vi "Add.vi"(6 "Options":T1={"DbType"=-1, "Direction"=-1, "Size"=-1, "Precision"=255, "Scale"=255} {"Direction" items=["Input"=1, "Output"=2, "InputOutput"=3, "ReturnValue"=6]; "DbType" items=["AnsiString"=0, "Binary"=1, "Byte"=2, "Boolean"=3, "Currency"=4, "Date"=5, "DateTime"=6, "Decimal"=7, "Double"=8, "Guid"=9, "Int16"=10, "Int32"=11, "Int64"=12, "Object"=13, "SByte"=14, "Single"=15, "String"=16, "Time"=17, "UInt16"=18, "UInt32"=19, "UInt64"=20, "VarNumeric"=21, "AnsiStringFixedLength"=22, "StringFixedLength"=23, "Xml"=25, "DateTime2"=26, "DateTimeOffset"=27]}, 8 "error in (no error)":errorcluster, 9 "value":variant, 10 "name":string, 11 "DynamicParameters in":refnum<class "DapperParameters.lvclass">) -> (0 "error out":errorcluster, 3 "DynamicParameters out":refnum<class "DapperParameters.lvclass">)   [LabVIEW 2020, in "ORM_Dapper.lvlib" / "DapperParameters.lvclass"]
uses:
  DapperParameters.lvclass
  System.Data
  DapperParameters.lvclass/DapperParameters.ctl
  C:/Viviota/Projects/R&D/__OpenSource/VIV_ORM/libraries/npgsql/System.Text.Json.dll
  libraries/npgsql/System.Text.Json.dll
  C:/Viviota/Projects/R&D/__OpenSource/VIV_ORM/libraries/dapper/Dapper.dll
  libraries/dapper/Dapper.dll
  Read ref.vi
  <vilib>/Viviota/shared/ORM.lvlibp/ORM/DynamicParameters/DynamicParameters.lvclass
  C:/Program Files/National Instruments/LabVIEW 2020/vi.lib/Viviota/shared/ORM.lvlibp/ORM/DynamicParameters/DynamicParameters.lvclass
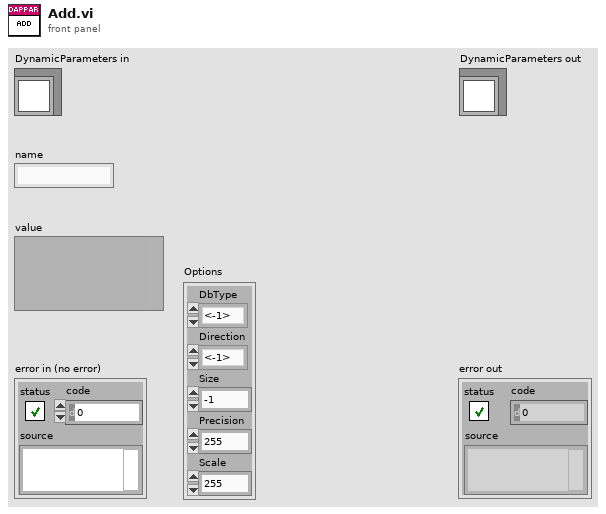
[diagram p1: front panel]
types:
  T1 = cluster{"DbType":i32, "Direction":i32, "Size":i32, "Precision":u8, "Scale":u8}
  T2 = typedef "ORM_Dapper.lvlib/dapper_dynamicparameters_ref.ctl" = refnum<k24>
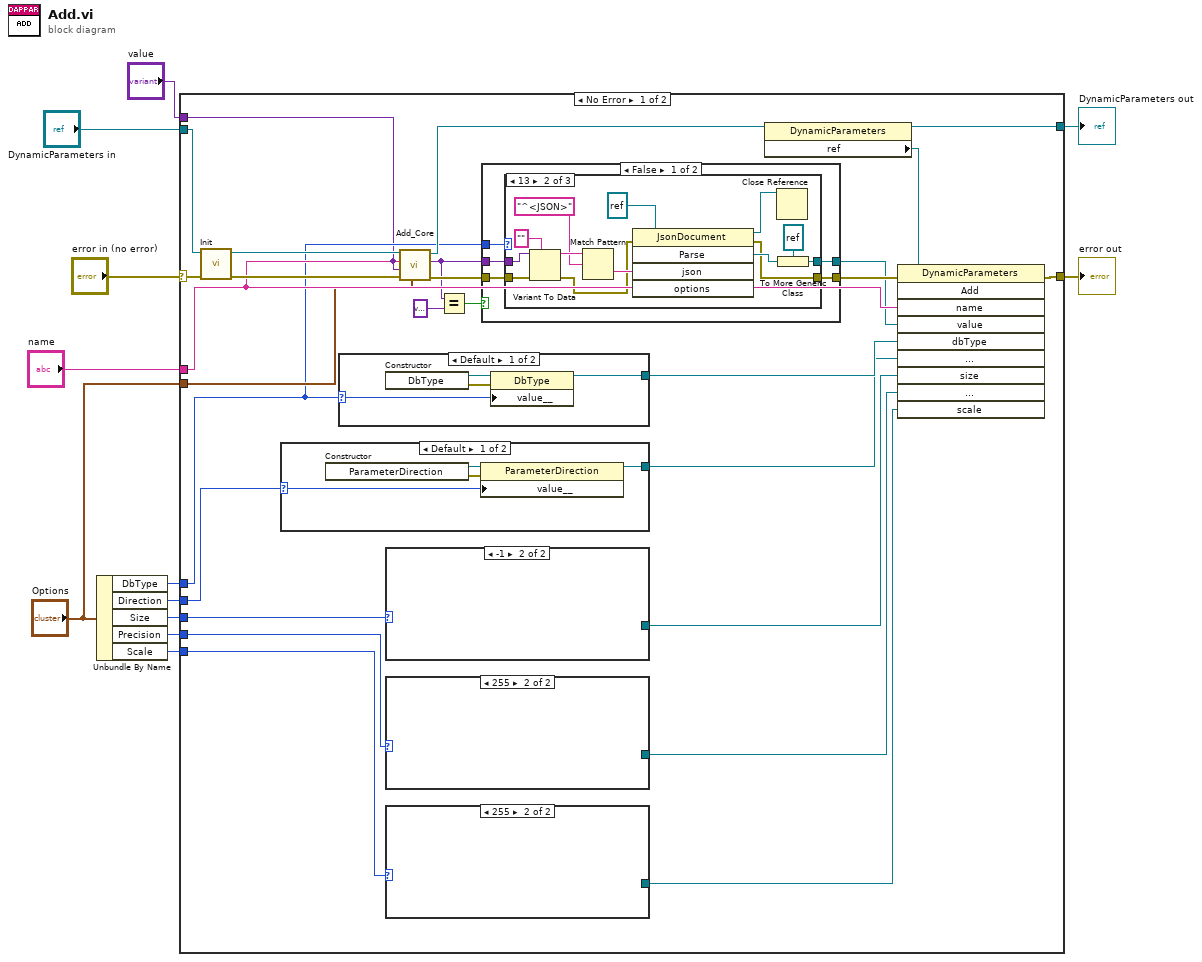
[diagram p0: block diagram]
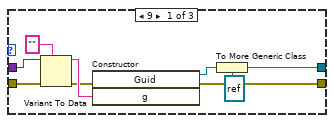
[diagram p2: hidden frame]
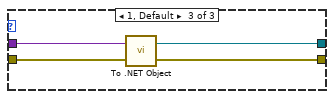
[diagram p3: hidden frame]
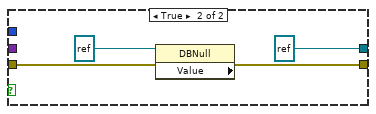
[diagram p4: hidden frame]
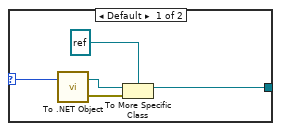
[diagram p5: hidden frame]
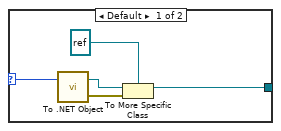
[diagram p7: hidden frame]
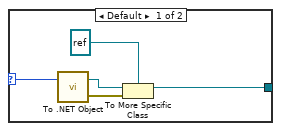
[diagram p9: hidden frame]
diagram:
  n1 = Unbundle By Name("Options") -> ("DbType"=w7:i32, "Direction"=w6:i32, "Size"=w5:i32, "Precision"=w4:u8, "Scale"=w3:u8)
  n2 = case shown="No Error" "error in (no error)" {
    selector: "error in (no error)" -> [w36 w97]
    tunnel: [w38 w97] -> w11
    tunnel: [w26 w96] -> w9
    tunnel: "DynamicParameters in" -> [w37 w96]
    tunnel: "name" -> [w21 _]
    tunnel: "value" -> [w15 _]
    tunnel: w6 -> [w34 _]
    tunnel: w3 -> [w33 _]
    tunnel: w4 -> [w31 _]
    tunnel: w7 -> [w16 _]
    tunnel: w5 -> [w28 _]
    tunnel: "Options" -> [w20 _]
    frame No Error {
      n3 = call "Init.vi"("error in (no error)"=w36, "DynamicParameters in"=w37) -> ("error out"=w24:errorcluster, "DynamicParameters out"=w23:refnum<class "DapperParameters.lvclass">)  [unwired: 8 in]
      n4 = case shown="Default" w34 {
        selector: w34 -> [w90 _]
        tunnel: [w89 _] -> w29
        frame Default {
          n5 = constructor class="ParameterDirection"() -> (reference out=w88:refnum<k24>, error out=w87:errorcluster)  [unwired: 3 in, 1 out]
          n6 = property class="ParameterDirection"(reference=w88, error in=w87, "value__"=w90) -> (reference out=w89:refnum<k24>)  [unwired: 1 out]
        }
        frame -1 {
        }
      }
      n7 = case shown="Default" w16 {
        selector: w16 -> [w81 _]
        tunnel: [w80 _] -> w30
        frame Default {
          n8 = constructor class="DbType"() -> (reference out=w79:refnum<k24>, error out=w78:errorcluster)  [unwired: 3 in, 1 out]
          n9 = property class="DbType"(reference=w79, error in=w78, "value__"=w81) -> (reference out=w80:refnum<k24>)  [unwired: 1 out]
        }
        frame -1 {
        }
      }
      n10 = case shown="-1" w28 {
        selector: w28 -> [w77 _]
        tunnel: [w75 _] -> w27
        frame Default {
          n11 = call <vilib>:"To .NET Object.vi"("anything"=w77) -> ("error out"=w73:errorcluster, ".NET object"=w76:refnum<k24>)  [unwired: 1 in]
          n12 = To More Specific Class(target class=refnum<k24> refnum ("size"), reference=w76, error in=w73) -> (specific class reference=w75:refnum<k24>)  [unwired: 1 out]
        }
        frame -1 {
        }
      }
      n13 = case shown="255" w31 {
        selector: w31 -> [w91 _]
        tunnel: [w92 _] -> w35
        frame Default {
          n14 = call <vilib>:"To .NET Object.vi"("anything"=w91) -> ("error out"=w95:errorcluster, ".NET object"=w93:refnum<k24>)  [unwired: 1 in]
          n15 = To More Specific Class(target class=refnum<k24> refnum ("size"), reference=w93, error in=w95) -> (specific class reference=w92:refnum<k24>)  [unwired: 1 out]
        }
        frame 255 {
        }
      }
      n16 = case shown="255" w33 {
        selector: w33 -> [w82 _]
        tunnel: [w83 _] -> w32
        frame Default {
          n17 = call <vilib>:"To .NET Object.vi"("anything"=w82) -> ("error out"=w84:errorcluster, ".NET object"=w86:refnum<k24>)  [unwired: 1 in]
          n18 = To More Specific Class(target class=refnum<k24> refnum ("size"), reference=w86, error in=w84) -> (specific class reference=w83:refnum<k24>)  [unwired: 1 out]
        }
        frame 255 {
        }
      }
      n19 = call <vilib>:"Add_Core.vi"("Options"=w20, "error in (no error)"=w24, "value"=w15, "name"=w21, "DynamicParameters in"=w23) -> ("error out"=w19:errorcluster, "DynamicParameters out"=w22:refnum<class "DapperParameters.lvclass">)  [unwired: 5 in]
      n20 = Equal?(x=w15, y=variant) -> (x = y?=w13:bool)
      n21 = case shown="False" w13 {
        tunnel: w19 -> [w43 w72]
        tunnel: [w42 w72] -> w18
        tunnel: [w41 refnum<k24> refnum (".NET object")] -> w17
        tunnel: w16 -> [w40 _]
        tunnel: w15 -> [w39 _]
        frame False {
          n22 = case shown="13" w40 {
            tunnel: [w45 w55 w66] -> w41
            tunnel: w43 -> [w52 w54 w69]
            tunnel: [w46 w56 w68] -> w42
            tunnel: w39 -> [w51 w53 w67]
            frame 9 {
              n23 = Variant To Data(error in=w52, type="", Variant=w51) -> (data=w49:string, error out=w48:errorcluster)
              n24 = constructor class="System.Guid" ("Constructor Node")(error in=w48, "g"=w49) -> (reference out=w47:refnum<k24>, error out=w46:errorcluster)  [unwired: 2 in, 2 out]
              n25 = To More Generic Class(target class=refnum<k24> refnum ("Value"), reference=w47) -> (generic class reference=w45:refnum<k24>)
            }
            frame 13 {
              n26 = Variant To Data(error in=w54, type="", Variant=w53) -> (data=w63:string, error out=w59:errorcluster)
              n27 = Match Pattern(string=w63, regular expression="^<JSON>") -> (after substring=w60:string)  [unwired: 1 in, 3 out]
              n28 = invoke class="JsonDocument" method="Parse"(reference=refnum<k24> refnum ("Value"), error in=w59, "json"=w60) -> (reference out=w57:refnum<k24>, error out=w56:errorcluster, "Parse"=w58:refnum<k24>)  [unwired: 2 in, 2 out]
              n29 = Close Reference(reference=w57) -> ()  [unwired: 1 in, 1 out]
              n30 = To More Generic Class(target class=refnum<k24> refnum ("Value"), reference=w58) -> (generic class reference=w55:refnum<k24>)
            }
            frame 1, Default {
              n31 = call <vilib>:"To .NET Object.vi"("error in (no error)"=w69, "anything"=w67) -> ("error out"=w68:errorcluster, ".NET object"=w66:refnum<k24>)
            }
          }
        }
        frame True {
          n32 = property class="DBNull" props=["Value"](reference=refnum<k24> refnum (".NET object")) -> ()  [unwired: 1 in, 3 out]
        }
      }
      n33 = property class="DynamicParameters"(reference=w22) -> (reference out=w26:refnum<class "DapperParameters.lvclass">, "ref"=w25:T2)  [unwired: 1 in, 1 out]
      n34 = invoke class="DynamicParameters" method="Add"(reference=w25, error in=w18, "name"=w21, "value"=w17, "dbType"=w30, "direction"=w29, "size"=w27, "precision"=w35, "scale"=w32) -> (error out=w38:errorcluster)  [unwired: 1 in, 9 out]
    }
    frame Error {
    }
  }
  "error out" <- w11
  "DynamicParameters out" <- w9
